vi "SS2 Live_Special Controls Update.vi"(7 "Verbose (T)":bool=TRUE, 8 "error in (no error)":errorcluster, 9 "Settings List Element":T1, 11 "VI Refnum":refnum<vi>) -> (0 "Error Out":errorcluster)   [LabVIEW 2019]
uses:
  SS2 Live_Settings List.ctl
  SS2 Live_Settings Q Element.ctl
  SS2 Live_Settings Q Action.ctl
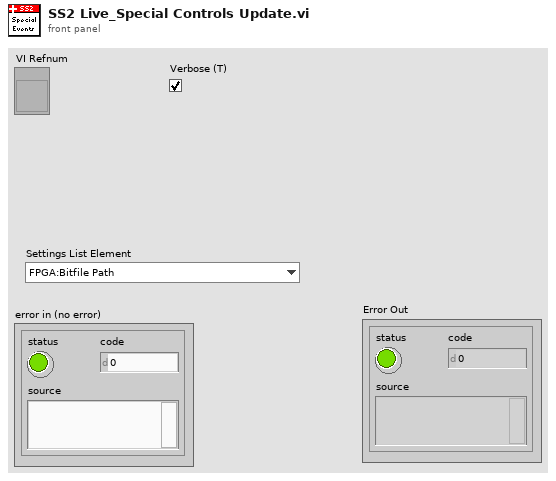
[diagram p1: front panel]
types:
  T1 = typedef "SS2 Live_Settings List.ctl" = enum16{"FPGA:Bitfile Path", "FPGA:Bitfile Version", "Acquisition Parameters:SS2 DAQ Parameters", "Acquisition Parameters:Gate Configuration Array", "Acquisition Parameters:Buffer Size (# Gates)", "File Information:File Information", "File Information:# Datasets in Series", "Image Parameters:Image ROI Information", "Image Parameters:Image Binning Options", "UI Parameters:Histogram Bins Number"}
  T2 = typedef "SS2 Live_Settings Q Element.ctl" = cluster{"Action":T3, "Data":variant}
  T3 = typedef "SS2 Live_Settings Q Action.ctl" = enum16{"Idle", "Store Current Configuration", "Rename Current Configuration", "Delete Current Configuration", "Update Image ROI Information", "Quit"}
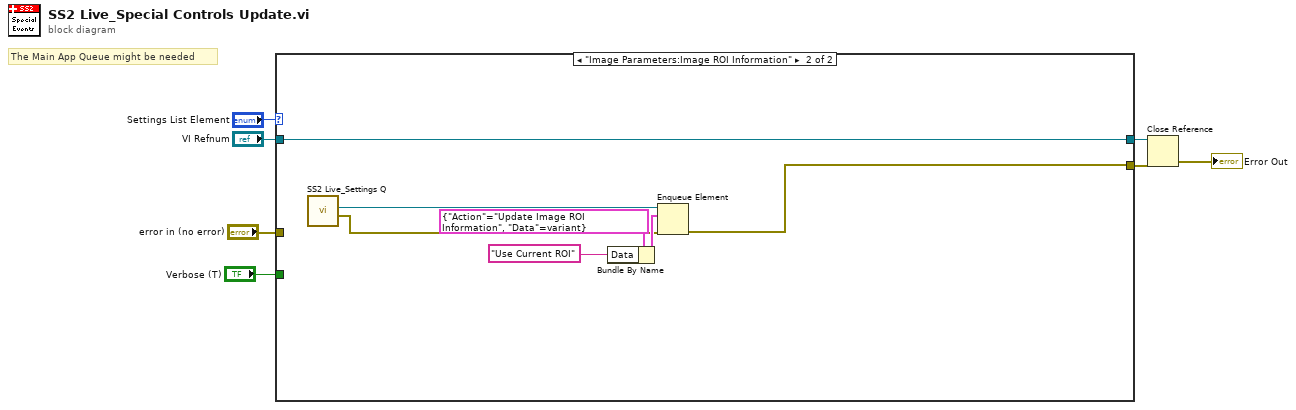
[diagram p0: block diagram]
diagram:
  # "The Main App Queue might be needed"
  n1 = case shown="\"Image Parameters:Image ROI Information\"" "Settings List Element" {
    tunnel: "VI Refnum" -> [w9 w16]
    tunnel: "error in (no error)" -> [w8 _]
    tunnel: [w9 w16] -> w4
    tunnel: [w8 w12] -> w2
    tunnel: "Verbose (T)" -> [_ _]
    frame "FPGA:Bitfile Path", Default {
    }
    frame "Image Parameters:Image ROI Information" {
      n2 = call "SS2 Live_Settings Q.vi"() -> ("error out"=w10:errorcluster, "Queue out"=w11:refnum<queue>)  [unwired: 10 in]
      n3 = Bundle By Name(cluster=T2 {"Action"=enum."Update Image ROI Information", "Data"=variant} ("element"), "Data"="Use Current ROI") -> (w14:T2)
      n4 = Enqueue Element(queue=w11, element=w14, error in (no error)=w10) -> (error out=w12:errorcluster)  [unwired: 1 in, 2 out]
    }
  }
  n5 = Close Reference(reference=w4, error in (no error)=w2) -> (error out=→"Error Out":errorcluster)
